vi "Write file.vi"(8 "error in (no error)":errorcluster, 11 "TomoConversion in":refnum<class "TomoConversion.lvclass">) -> (0 "error out":errorcluster, 3 "TomoConversion out":refnum<class "TomoConversion.lvclass">)   [LabVIEW 2012, in "TomoConversion.lvclass"]
uses:
  TomoConversion.lvclass
  TomoConversion.lvclass/TomoConversion.ctl
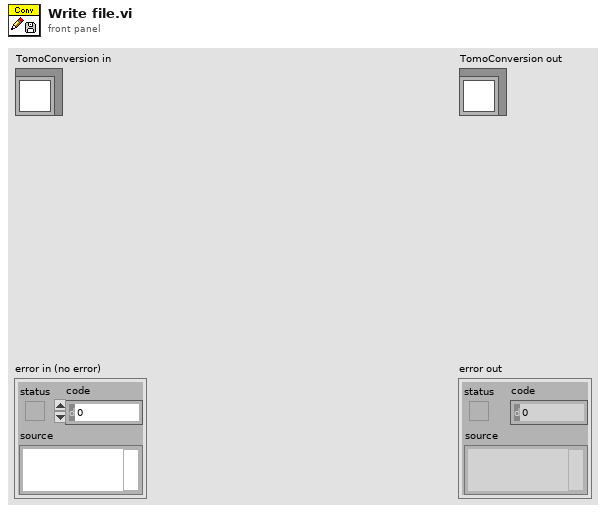
[diagram p1: front panel]
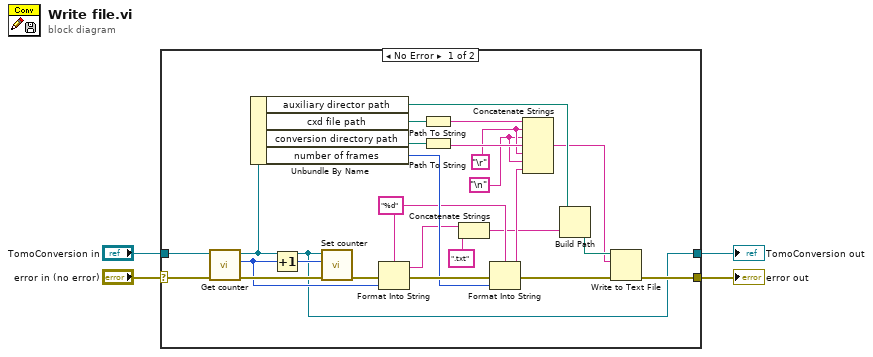
[diagram p0: block diagram]
diagram:
  n1 = case shown="No Error" "error in (no error)" {
    selector: "error in (no error)" -> [w29 w31]
    tunnel: [w10 w31] -> w3
    tunnel: [w9 w30] -> w1
    tunnel: "TomoConversion in" -> [w28 w30]
    frame No Error {
      w14 = "%d" ("format string")
      w16 = "\n"
      w17 = "\r"
      n2 = call-dynamic "Get counter.vi"("error in (no error)"=w29, "TomoConversion in"=w28) -> ("error out"=w27:errorcluster, "counter"=w23:u32, "TomoConversion out"=w9:refnum<class "TomoConversion.lvclass">)  [unwired: 7 in]
      n3 = Unbundle By Name(w9) -> ("auxiliary director path"=w13:path, "cxd file path"=w21:path, "conversion directory path"=w20:path, "number of frames"=w22:i32)
      n4 = Increment(x=w23) -> (x+1=w26:u32)
      n5 = call-dynamic "Set counter.vi"("error in (no error)"=w27, "counter"=w26, "TomoConversion in"=w9) -> ("error out"=w25:errorcluster)  [unwired: 7 in, 1 out]
      n6 = Format Into String(format string=w14, error in=w25, w23) -> (resulting string=w8:string, error out=w24:errorcluster)  [unwired: 1 in]
      n7 = Path To String(path=w21) -> (string=w19:string)
      n8 = Path To String(path=w20) -> (string=w18:string)
      n9 = Concatenate Strings(w8, ".txt" ("format string")) -> (w7:string)
      n10 = Format Into String(format string=w14, error in=w24, w22) -> (resulting string=w15:string, error out=w12:errorcluster)  [unwired: 1 in]
      n11 = Concatenate Strings(w19, w17, w16, w18, w17, w16, w15) -> (w5:string)
      n12 = Build Path(base path=w13, name or relative path=w7) -> (appended path=w11:path)
      n13 = Write to Text File(file (use dialog)=w11, text=w5, error in=w12) -> (error out=w10:errorcluster)  [unwired: 1 in, 2 out]
    }
    frame Error {
    }
  }
  "error out" <- w3
  "TomoConversion out" <- w1
